vi "Load Config.vi"() -> (3 "Array":T3(array[cluster]))   [LabVIEW 2019, in "LINX.lvlib" / "LINX.lvclass"]
uses:
  LINX.lvclass
  LINX Shortcut.ctl
  LINX Channel Type.ctl
  <vilib>/Utility/config.llb/Read Key (String).vi
  <vilib>/Utility/config.llb/Read Key (I32).vi
  <vilib>/Utility/config.llb/NI_LVConfig.lvlib
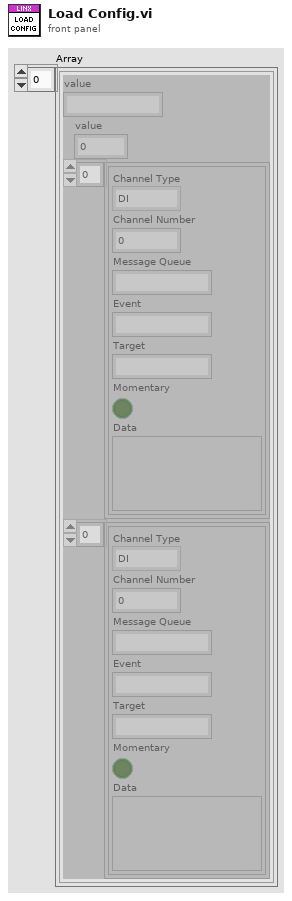
[diagram p1: front panel]
types:
  T1 = typedef "LINX.lvlib/LINX.lvclass/LINX Shortcut.ctl" = cluster{"Channel Type":T2, "Channel Number":u8, "Message Queue":string, "Event":string, "Target":string, "Momentary":bool, "Data":variant}
  T2 = typedef "LINX.lvlib/LINX.lvclass/LINX Channel Type.ctl" = enum16{"DI", "AI"}
  T3 = cluster{"value":string, "value":i32, T1[], T1[]}[]
  T4 = typedef "NI_LVConfig.lvlib/Config Data RefNum.ctl" = refnum<k1>
  T5 = cluster{string, "Message Queue":string, "Event":string, "Target":string, "Momentary":bool, "Data":variant}
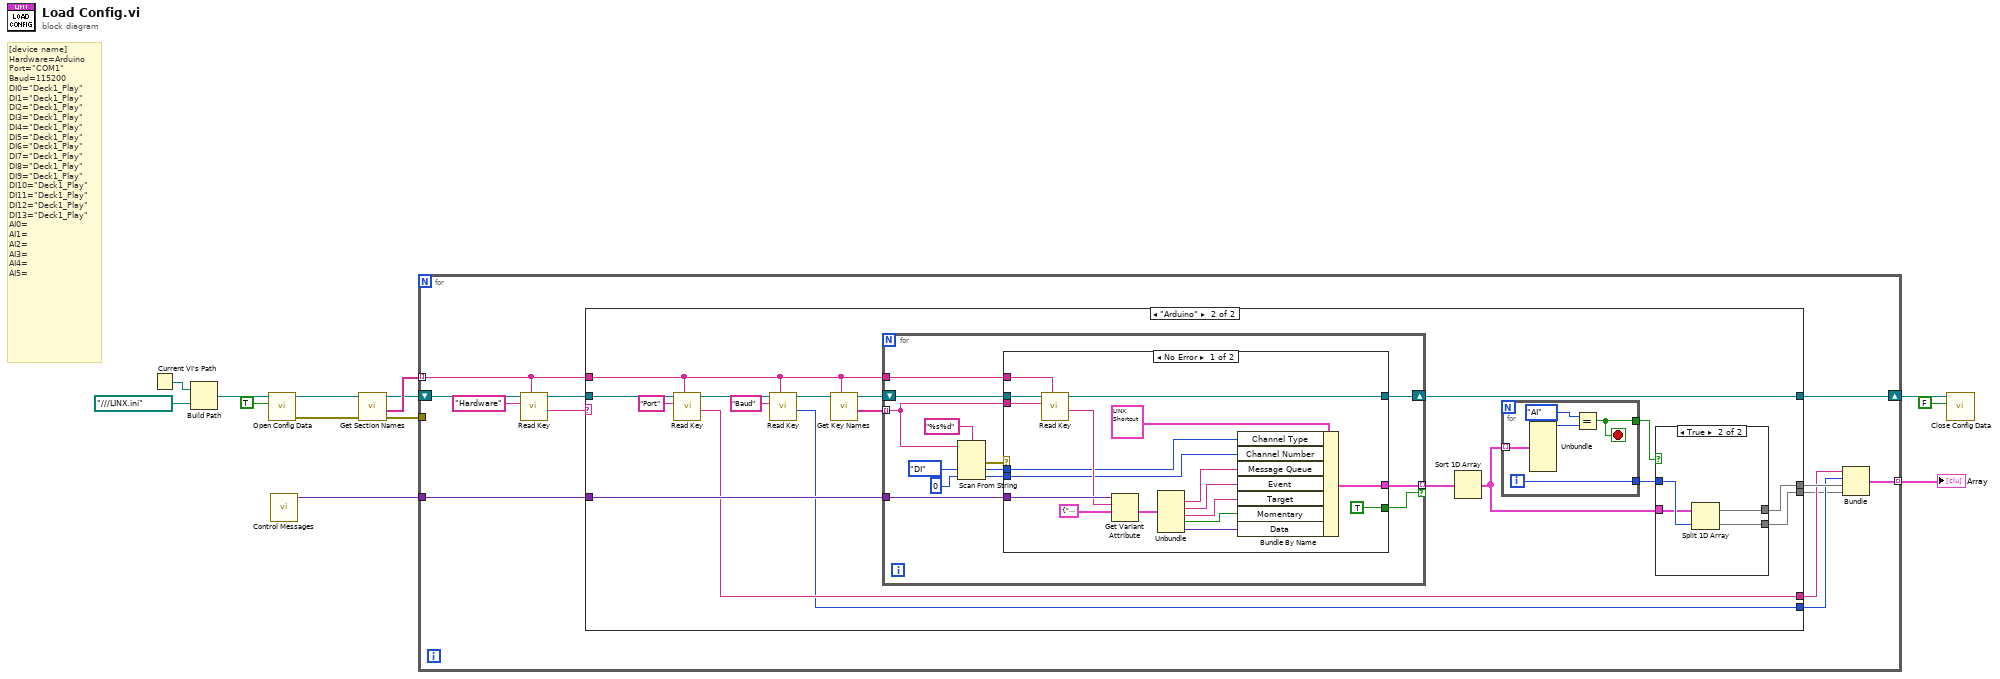
[diagram p0: block diagram]
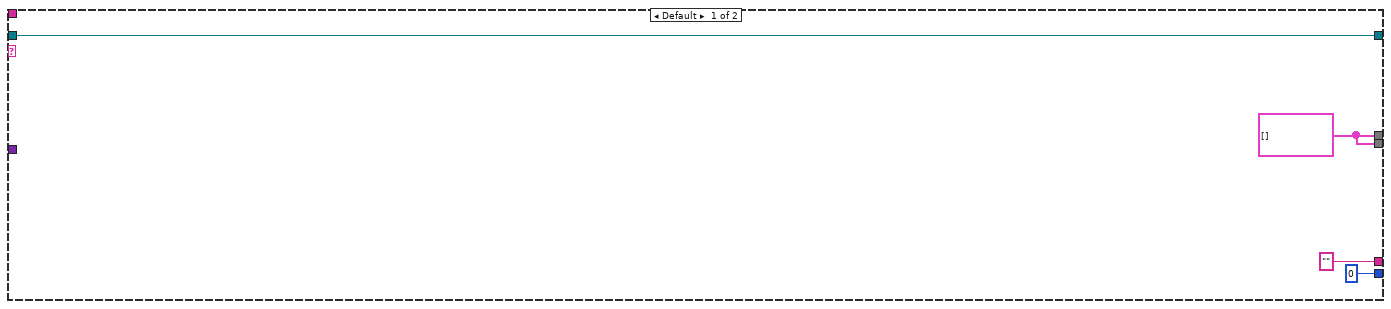
[diagram p2: hidden frame]
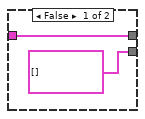
[diagram p3: hidden frame]
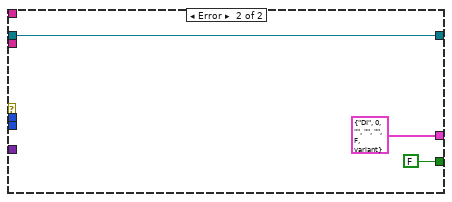
[diagram p4: hidden frame]
diagram:
  # "[device name]\nHardware=Arduino\nPort=\"COM1\"\nBaud=115200\nDI0=\"Deck1_Play\"\nDI1=\"Deck1_Play\"\nDI2=\"Deck1_Play\"\nDI3=\"Deck1_Play\"\nDI4=\"Deck1_Play\"\nDI5=\"Deck1_Play\"\nDI6=\"Deck1_Play\"\nDI7=\"Deck1_Play\"\nDI8=\"Deck1_Play\"\nDI9=\"Deck1_Play\"\nDI10=\"Deck1_Play\"\nDI11=\"Deck1_Play\"\nDI12=\"Deck1_Play\"\nDI13=\"Deck1_Play\"\nAI0=\nAI1=\nAI2=\nAI3=\nAI4=\nAI5="
  n1 = Current VI's Path() -> (path=w3:path)
  n2 = Build Path(base path=w3, name or relative path=path "../../../LINX.ini" ("configuration file path")) -> (appended path=w1:path)
  n3 = call <vilib>:"Open Config Data.vi"("create file if necessary (T)"=TRUE, "configuration file path"=w1) -> ("error out"=w11:errorcluster, "refnum"=w12:T4)  [unwired: 7 in, 1 out]
  n4 = call "Control Messages.vi"() -> ("Shortcuts"=w10:variant)  [unwired: 11 in]
  n5 = call <vilib>:"Get Section Names.vi"("error in (no error)"=w11, "refnum"=w12) -> ("error out"=w7:errorcluster, "section names"=w9:string[], "refnum out"=w8:T4)  [unwired: 7 in]
  n6 = for {
    tunnel: w9 -> [w21] mode=indexing
    tunnel: w7 -> [_]
    shift-right: [w19] -> w5
    shift-left: w8 -> [w25]
    tunnel: w10 -> [w20]
    tunnel: [w17] -> w6 mode=indexing
    n7 = call-poly <vilib>:"Read Key.vi"("section"=w21, "key"="Hardware", "refnum"=w25) -> ("value"=w23:string, "refnum out"=w22:T4)  [unwired: 5 in, 2 out]
    n8 = case shown="\"Arduino\"" w23 {
      tunnel: w22 -> [w29 w47]
      tunnel: w21 -> [_ w40]
      tunnel: w20 -> [_ w39]
      tunnel: [w29 w37] -> w19
      tunnel: [w28 w31] -> w18
      tunnel: ["" ("value") w36] -> w16
      tunnel: [0 ("value") w35] -> w15
      tunnel: [w28 w30] -> w14
      frame Default {
        w28 = T1[] []
      }
      frame "Arduino" {
        n9 = call-poly <vilib>:"Read Key.vi"("section"=w40, "key"="Port", "refnum"=w47) -> ("value"=w36:string, "refnum out"=w45:T4)  [unwired: 5 in, 2 out]
        n10 = call-poly <vilib>:"Read Key.vi"("section"=w40, "key"="Baud", "refnum"=w45) -> ("value"=w35:i32, "refnum out"=w43:T4)  [unwired: 5 in, 2 out]
        n11 = call <vilib>:"Get Key Names.vi"("section"=w40, "refnum"=w43) -> ("key names"=w42:string[], "refnum out"=w41:T4)  [unwired: 6 in, 2 out]
        n12 = for {
          tunnel: w42 -> [w68] mode=indexing
          shift-right: [w69] -> w37
          shift-left: w41 -> [w70]
          tunnel: w40 -> [w63]
          tunnel: w39 -> [w62]
          tunnel: [w60] -> w38 mode=indexing if=w59
          n13 = Scan From String(format string="%s%d", input string=w68, default 1=LINX_Channel_Type."DI" ("Channel Type"), default 2=u8 0 ("default value 2")) -> (error out=w66:errorcluster, output 1=w65:T2, output 2=w64:u8)  [unwired: 2 in, 2 out]
          n14 = case shown="No Error" w66 {
            tunnel: w70 -> [w89 w91]
            tunnel: [w88 w91] -> w69
            tunnel: w68 -> [w87 _]
            tunnel: w65 -> [w80 _]
            tunnel: w64 -> [w79 _]
            tunnel: w63 -> [w86 _]
            tunnel: w62 -> [w85 _]
            tunnel: [w73 T1 {"Channel Type"=enum."DI", "Channel Number"=0, "Message Queue"="", "Event"="", "Target"="", "Momentary"=FALSE, "Data"=variant} ("DAQmx Shortcut")] -> w60
            tunnel: [TRUE FALSE] -> w59
            frame No Error {
              n15 = call-poly <vilib>:"Read Key.vi"("section"=w86, "key"=w87, "refnum"=w89) -> ("value"=w84:string, "refnum out"=w88:T4)  [unwired: 5 in, 2 out]
              n16 = Get Variant Attribute(Variant=w85, name=w84, default value (empty Variant)=T5 {"", "Message Queue"="", "Event"="", "Target"="", "Momentary"=FALSE, "Data"=variant} ("DAQmx Shortcut")) -> (value=w81:T5)  [unwired: 1 in, 3 out]
              n17 = Unbundle(w81) -> ("Message Queue"=w78:string, "Event"=w77:string, "Target"=w76:string, "Momentary"=w75:bool, "Data"=w74:variant)  [unwired: 1 out]
              n18 = Bundle By Name(cluster=T1 {"Channel Type"=enum."AI", "Channel Number"=0, "Message Queue"="Mixer", "Event"="Value Change", "Target"="Crossfader", "Momentary"=FALSE, "Data"=variant} ("DAQmx Shortcut"), "Channel Type"=w80, "Channel Number"=w79, "Message Queue"=w78, "Event"=w77, "Target"=w76, "Momentary"=w75, "Data"=w74) -> (w73:T1)
            }
            frame Error {
            }
          }
        }
        n19 = Sort 1D Array(array=w38) -> (sorted array=w32:T1[])
        n20 = for {
          tunnel: w32 -> [w58] mode=indexing
          tunnel: [w55] -> w33
          tunnel: [w54] -> w34
          i -> [w55]
          stop <- w54 stop-if-true
          n21 = Unbundle(w58) -> ("Channel Type"=w57:T2)  [unwired: 6 out]
          n22 = Equal?(x=LINX_Channel_Type."AI", y=w57) -> (x = y?=w54:bool)
        }
        n23 = case shown="True" w34 {
          tunnel: w33 -> [_ w53]
          tunnel: w32 -> [w49 w52]
          tunnel: [w49 w51] -> w31
          tunnel: [T1[] [] w50] -> w30
          frame False {
          }
          frame True {
            n24 = Split 1D Array(array=w52, index=w53) -> (first subarray=w51:T1[], second subarray=w50:T1[])
          }
        }
      }
    }
    n25 = Bundle("value"=w16, "value"=w15, w18, w14) -> (w17:cluster{"value":string, "value":i32, T1[], T1[]})  [unwired: 1 in]
  }
  "Array" <- w6
  n26 = call <vilib>:"Close Config Data.vi"("write file if changed (T)"=FALSE, "refnum"=w5) -> ()  [unwired: 8 in, 2 out]
